vi "StressDist_equivalent_calc.vi"(2 "Angle":dbl, 3 "Parameters":dbl[](array[numeric])) -> (0 "Stress":dbl)   [LabVIEW 2016]
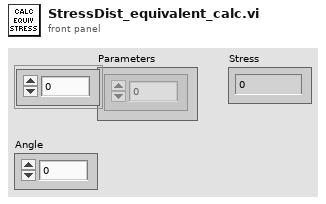
[diagram p1: front panel]
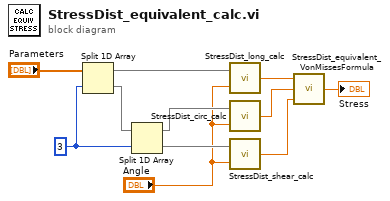
[diagram p0: block diagram]
diagram:
  w10 = 3 ("index")
  n1 = Split 1D Array(array="Parameters", index=w10) -> (first subarray=w8:dbl[], second subarray=w9:dbl[])
  n2 = Split 1D Array(array=w9, index=w10) -> (first subarray=w6:dbl[], second subarray=w7:dbl[])
  n3 = call "StressDist_long_calc.vi"("Angle"="Angle", "Parameters"=w8) -> ("Stress"=w5:dbl)
  n4 = call "StressDist_circ_calc.vi"("Angle"="Angle", "Parameters"=w6) -> ("Stress"=w3:dbl)
  n5 = call "StressDist_shear_calc.vi"("Angle"="Angle", "Parameters"=w7) -> ("Stress"=w2:dbl)
  n6 = call "StressDist_equivalent_VonMissesFormula.vi"("Sshear"=w2, "Scirc"=w3, "Slong"=w5) -> ("Sequi"=→"Stress":dbl)
